vi "Position Button Underneath.vi"(8 "error in (no error)":errorcluster, 10 "Flight Mode Ref":refnum<vi>, 11 "Button Ref":refnum<vi>) -> (0 "error out":errorcluster)   [LabVIEW 2014]
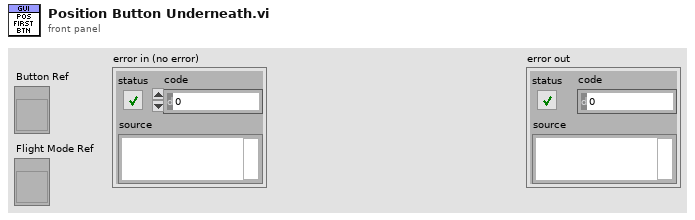
[diagram p1: front panel]
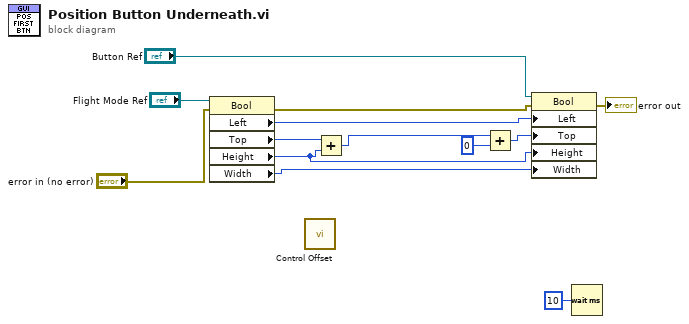
[diagram p0: block diagram]
diagram:
  n1 = property class="Bool"(reference="Flight Mode Ref", error in="error in (no error)") -> (error out=w12:errorcluster, "Left"=w8:i32, "Top"=w7:i32, "Height"=w4:u32, "Width"=w3:u32)  [unwired: 1 out]
  n2 = call "Control Offset.vi"() -> ()  [unwired: 11 in, 1 out]
  n3 = Add(x=w7, y=w4) -> (x+y=w6:u32)
  n4 = Add(x=w6, y=u32 0) -> (x+y=w9:u32)
  n5 = property class="Bool"(reference="Button Ref", error in=w12, "Left"=w8, "Top"=w9, "Height"=w4, "Width"=w3) -> (error out=→"error out":errorcluster)  [unwired: 1 out]
  n6 = Wait (ms)(milliseconds to wait=u32 10) -> ()  [unwired: 1 out]
